vi "Timer FGV.vi"(8 "Error In":errorcluster, 10 "Time Target (s)":dbl format="%#_13g", 11 "Timer state":enum16{"Reset", "Read", "Pause"}(ring)) -> (0 "Error Out":errorcluster, 2 "Time Elapsed?":bool, 3 "Elapsed Time":dbl)   [LabVIEW 2024]
doc: "This is the timer fgv. The VI calculate the dt and sum it up to calculate the total elapsed time.\n\nThe elapsed time is checked with target time and output the value"
panel:
  # "Outputs to the VI"
  # "Inputs to the VI"
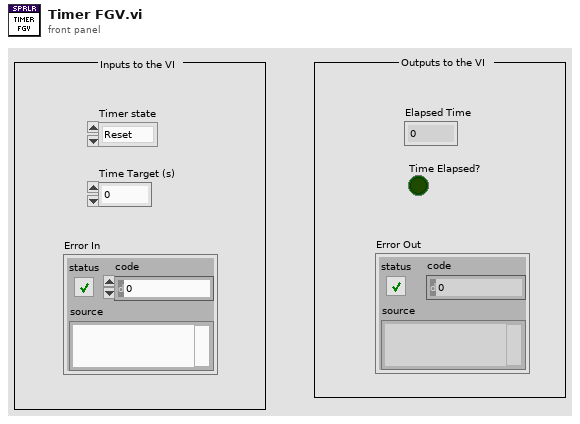
[diagram p1: front panel]
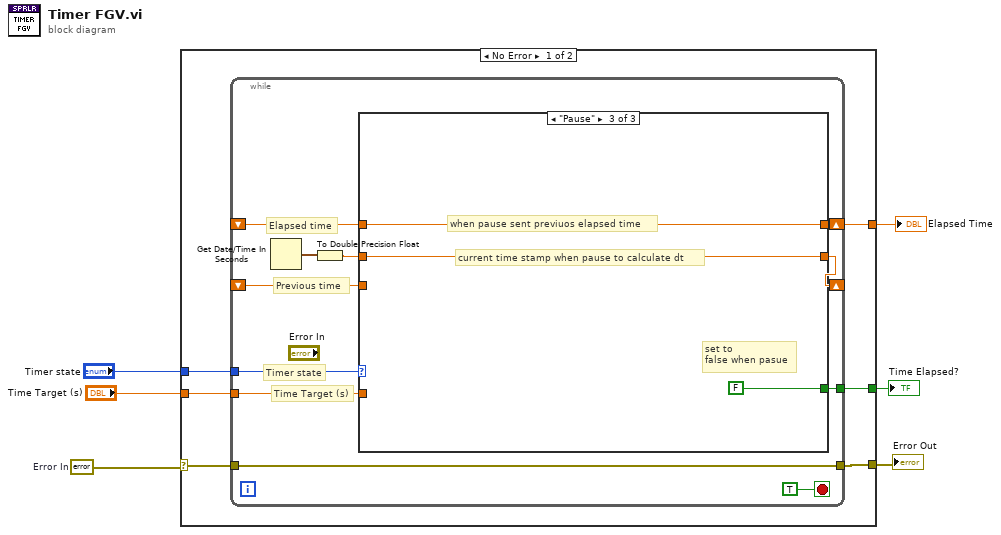
[diagram p0: block diagram]
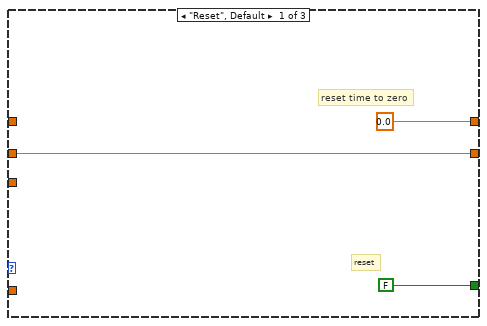
[diagram p2: hidden frame]
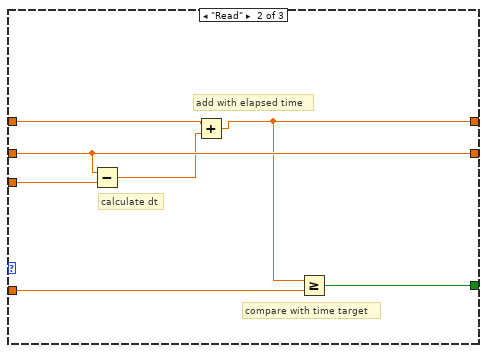
[diagram p3: hidden frame]
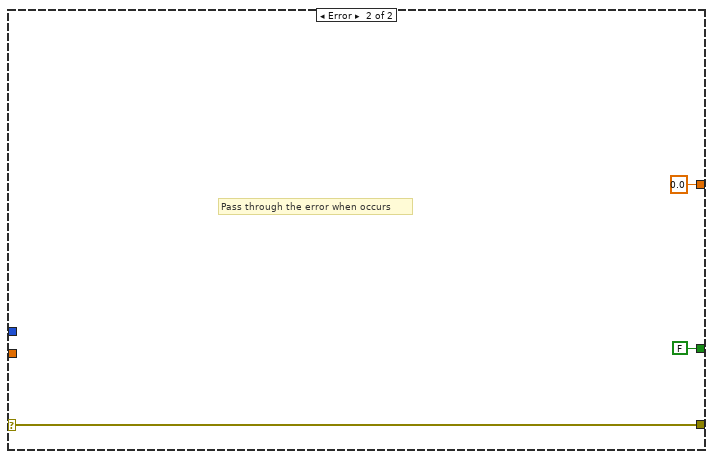
[diagram p4: hidden frame]
diagram:
  w6 = errorcluster {"status"=FALSE, "code"=0, "source"=""}  # Error In
  n1 = case shown="No Error" w6 {
    selector: w6 -> [w12 w38]
    tunnel: [w11 w38] -> w5
    tunnel: "Timer state" -> [w10 _]
    tunnel: [w9 0.0] -> w3
    tunnel: "Time Target (s)" -> [w8 _]
    tunnel: [w7 FALSE] -> w1
    frame No Error {
      n2 = while {
        tunnel: [w23] -> w11
        tunnel: w12 -> [w23]
        tunnel: w10 -> [w22]
        shift-right: [w18] -> _
        shift-left: _ -> [w19]
        shift-right: [w16] -> w9
        shift-left: _ -> [w17]
        tunnel: w8 -> [w15]
        tunnel: [w14] -> w7
        stop <- TRUE stop-if-true
        # "Previous time"
        # "Elapsed time"
        # "Time Target (s)"
        # "Timer state"
        n3 = Get Date/Time In Seconds() -> (seconds since 1Jan1904=w21:timestamp)
        n4 = To Double Precision Float(number=w21) -> (double precision float=w20:dbl)
        n5 = case shown="\"Pause\"" w22 {
          tunnel: w20 -> [w24 w32 w36]
          tunnel: w19 -> [_ w33 _]
          tunnel: [w24 w32 w36] -> w18
          tunnel: w17 -> [_ w30 w35]
          tunnel: [0.0 w28 w35] -> w16
          tunnel: w15 -> [_ w29 _]
          tunnel: [FALSE w27 FALSE] -> w14
          frame "Reset", Default {
            # "reset"
            # "reset time to zero"
          }
          frame "Read" {
            # "compare with time target"
            # "add with elapsed time"
            # "calculate dt"
            n6 = Subtract(x=w32, y=w33) -> (x-y=w31:dbl)
            n7 = Add(x=w30, y=w31) -> (x+y=w28:dbl)
            n8 = Greater Or Equal?(x=w28, y=w29) -> (x >= y?=w27:bool)
          }
          frame "Pause" {
            # "set to\nfalse when pasue"
            # "current time stamp when pause to calculate dt"
            # "when pause sent previuos elapsed time"
          }
        }
      }
    }
    frame Error {
      # "Pass through the error when occurs"
    }
  }
  "Error Out" <- w5
  "Elapsed Time" <- w3
  "Time Elapsed?" <- w1
